vi "Day08-sets_to_map.vi"(11 "Array of sets":set{u8}[](array[numeric])) -> (2 "map":map{u8, string}(c390))   [LabVIEW 2021]
uses:
  d25deb60-6f57-4a06-ae0f-7af60e17bb11.vi
  6c144e05-113f-4abc-a946-dcc71dd16d2c.vi
  50885f48-3acf-425f-b691-2fff5a063f99.vi
  a4c1d64e-348d-4501-935c-61f915fd6d8c.vi
  e3c87640-8722-4108-b74f-693c7f5a895b.vi
  e24fa3c4-d2f5-4d74-bc71-a5a6f3e85988.vi
  ecf9f81b-b63f-4c67-a316-a17628bb9b65.vi
  b5ef73c6-721d-49a5-af8d-99b87a8c5e20.vi
  a61a933c-3d81-4125-b1af-a12765048eee.vi
  9180e893-9a55-4de2-912c-ba3462fb0cb1.vi
  d947758a-7877-4e86-8535-d8998e87c975.vi
  741c12e9-90d2-4b95-9289-990daeb08a46.vi
  f7f2cf37-8755-47ea-a3f2-be66d21816cf.vi
  0f8ddcea-e4d1-45d8-b5ed-1b510dd1aaf7.vi
  e392e3a7-f24e-4884-bbbe-f5b43754e05e.vi
  d2f13c56-e0e9-48d2-b6df-c4eb8dad29bd.vi
  76191552-7462-44bb-8eb7-dfd9036bbebb.vi
panel:
  out "c":u8
  out "f":u8
  out "e":u8
  out "g":u8
  out "b":u8
  out "d":u8
  out "a":u8
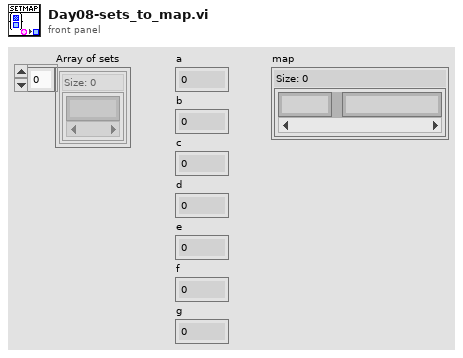
[diagram p1: front panel]
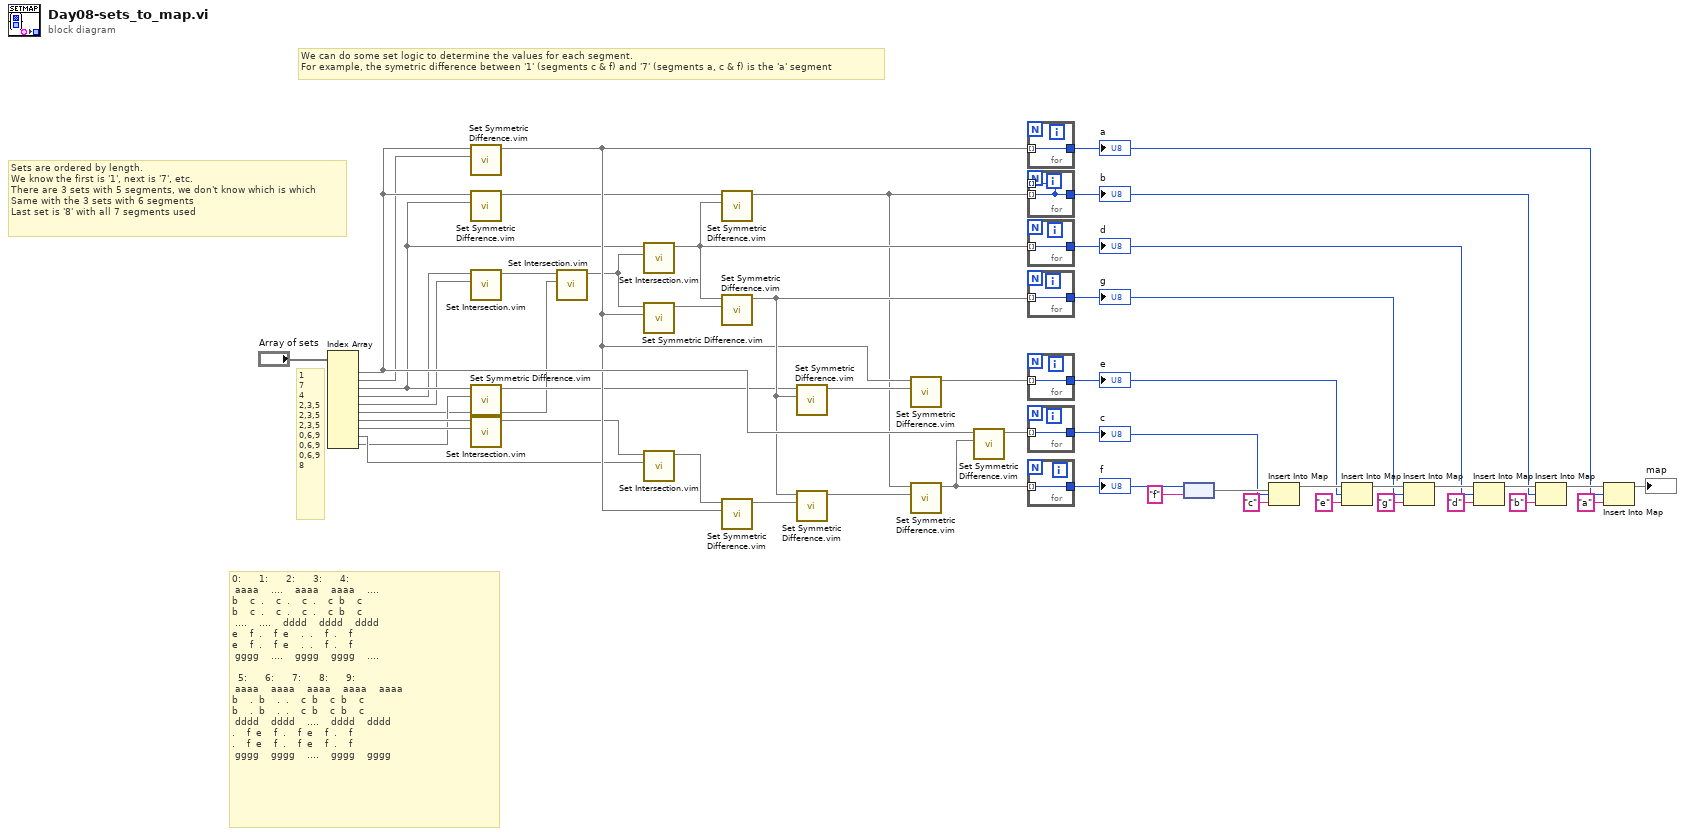
[diagram p0: block diagram]
diagram:
  # "We can do some set logic to determine the values for each segment.\nFor example, the symetric difference between '1' (segments c & f) and '7' (segments a, c & f) is the 'a' segment"
  # "0:      1:      2:      3:      4:\n aaaa    ....    aaaa    aaaa    ....\nb    c  .    c  .    c  .    c  b    c\nb    c  .    c  .    c  .    c  b    c\n ....    ....    dddd    dddd    dddd\ne    f  .    f  e    .  .    f  .    f\ne    f  .    f  e    .  .    f  .    f\n gggg    ....    gggg    gggg    ....\n\n  5:      6:      7:      8:      9:\n aaaa    aaaa    aaaa    aaaa    aaaa\nb    .  b    .  .    c  b    c  b    c\nb    .  b    .  .    c  b    c  b    c\n dddd    dddd    ....    dddd    dddd\n.    f  e    f  .    f  e    f  .    f\n.    f  e    f  .    f  e    f  .    f\n gggg    gggg    ....    gggg    gggg"
  # "Sets are ordered by length.\nWe know the first is '1', next is '7', etc.\nThere are 3 sets with 5 segments, we don't know which is which\nSame with the 3 sets with 6 segments\nLast set is '8' with all 7 segments used"
  # "1\n7\n4\n2,3,5\n2,3,5\n2,3,5\n0,6,9\n0,6,9\n0,6,9\n8"
  n1 = Index Array(array="Array of sets") -> (element #1=w34:set{u8}, element #2=w11:set{u8}, element #3=w22:set{u8}, element #4=w19:set{u8}, element #5=w12:set{u8}, element #6=w13:set{u8}, element #7=w24:set{u8}, element #8=w25:set{u8}, element #9=w27:set{u8}, element #10=w18:set{u8})  [unwired: 10 in]
  n2 = call "Set Symmetric Difference.vim"("set 2"=w11, "set 1"=w34) -> ("symmetric difference"=w29:set{u8})  [unwired: 9 in]
  n3 = call "Set Symmetric Difference.vim"("set 2"=w22, "set 1"=w34) -> ("symmetric difference"=w14:set{u8})  [unwired: 9 in]
  n4 = call "Set Intersection.vim"("set 2"=w12, "set 1"=w19) -> ("intersection"=w9:set{u8})  [unwired: 9 in]
  n5 = call "Set Symmetric Difference.vim"("set 2"=w18, "set 1"=w22) -> ("symmetric difference"=w20:set{u8})  [unwired: 9 in]
  n6 = call "Set Intersection.vim"("set 2"=w25, "set 1"=w24) -> ("intersection"=w26:set{u8})  [unwired: 9 in]
  n7 = call "Set Intersection.vim"("set 2"=w13, "set 1"=w9) -> ("intersection"=w15:set{u8})  [unwired: 9 in]
  n8 = call "Set Intersection.vim"("set 2"=w15, "set 1"=w22) -> ("intersection"=w17:set{u8})  [unwired: 9 in]
  n9 = call "Set Symmetric Difference.vim"("set 2"=w29, "set 1"=w15) -> ("symmetric difference"=w16:set{u8})  [unwired: 9 in]
  n10 = call "Set Intersection.vim"("set 2"=w27, "set 1"=w26) -> ("intersection"=w28:set{u8})  [unwired: 9 in]
  n11 = call "Set Symmetric Difference.vim"("set 2"=w17, "set 1"=w14) -> ("symmetric difference"=w8:set{u8})  [unwired: 9 in]
  n12 = call "Set Symmetric Difference.vim"("set 2"=w16, "set 1"=w17) -> ("symmetric difference"=w31:set{u8})  [unwired: 9 in]
  n13 = call "Set Symmetric Difference.vim"("set 2"=w29, "set 1"=w28) -> ("symmetric difference"=w30:set{u8})  [unwired: 9 in]
  n14 = call "Set Symmetric Difference.vim"("set 2"=w31, "set 1"=w20) -> ("symmetric difference"=w21:set{u8})  [unwired: 9 in]
  n15 = call "Set Symmetric Difference.vim"("set 2"=w30, "set 1"=w31) -> ("symmetric difference"=w32:set{u8})  [unwired: 9 in]
  n16 = call "Set Symmetric Difference.vim"("set 2"=w21, "set 1"=w29) -> ("symmetric difference"=w23:set{u8})  [unwired: 9 in]
  n17 = call "Set Symmetric Difference.vim"("set 2"=w32, "set 1"=w8) -> ("symmetric difference"=w33:set{u8})  [unwired: 9 in]
  n18 = call "Set Symmetric Difference.vim"("set 2"=w33, "set 1"=w34) -> ("symmetric difference"=w35:set{u8})  [unwired: 9 in]
  n19 = for {
    tunnel: [w50] -> w1
    tunnel: w29 -> [w50] mode=indexing
  }
  "a" <- w1
  n20 = for {
    tunnel: [w51] -> w2
    tunnel: [w51] -> _ mode=indexing
    tunnel: w8 -> [w51] mode=indexing
  }
  "b" <- w2
  n21 = for {
    tunnel: [w52] -> w3
    tunnel: w17 -> [w52] mode=indexing
  }
  "d" <- w3
  n22 = for {
    tunnel: [w53] -> w4
    tunnel: w31 -> [w53] mode=indexing
  }
  "g" <- w4
  n23 = for {
    tunnel: [w54] -> w5
    tunnel: w23 -> [w54] mode=indexing
  }
  "e" <- w5
  n24 = for {
    tunnel: [w55] -> w6
    tunnel: w35 -> [w55] mode=indexing
  }
  "c" <- w6
  n25 = for {
    tunnel: [w56] -> w7
    tunnel: w33 -> [w56] mode=indexing
  }
  "f" <- w7
  n26 = node(w7, "f") -> (w37:map{u8, string})
  n27 = Insert Into Map(map in=w37, key=w6, value="c") -> (map out=w39:map{u8, string})  [unwired: 2 out]
  n28 = Insert Into Map(map in=w39, key=w5, value="e") -> (map out=w40:map{u8, string})  [unwired: 2 out]
  n29 = Insert Into Map(map in=w40, key=w4, value="g") -> (map out=w41:map{u8, string})  [unwired: 2 out]
  n30 = Insert Into Map(map in=w41, key=w3, value="d") -> (map out=w42:map{u8, string})  [unwired: 2 out]
  n31 = Insert Into Map(map in=w42, key=w2, value="b") -> (map out=w47:map{u8, string})  [unwired: 2 out]
  n32 = Insert Into Map(map in=w47, key=w1, value="a") -> (map out=→"map":map{u8, string})  [unwired: 2 out]
